vi "FGV Map of Errors.vi"(7 "Operation (Get)":enum16{"Init", "Get", "Update"}(ring)=enum."Get", 8 "error in":errorcluster, 10 "error description":string, 11 "error code":i32) -> (0 "error out":errorcluster, 3 "Custom Errors out":map{i32, string}(c390))   [LabVIEW 2021]
doc: "FGV storing <b>Custom Errors</b> values. Initialize the map by Init <b>Operation</b>, access the map by Get (default) or update the map by selecting Update <b>Operation</b> and wire <b>error code</b> as a key and <b>error description</b> as a value."
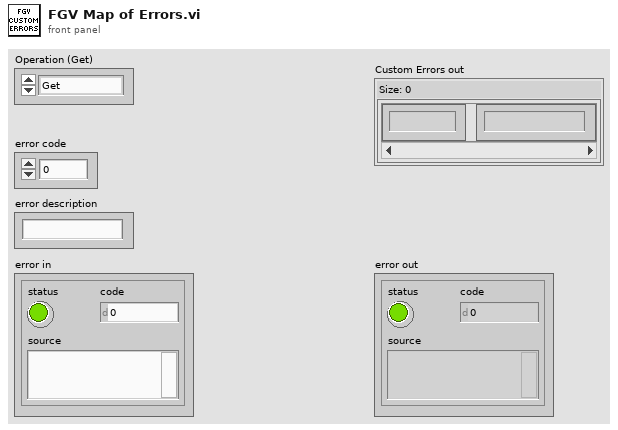
[diagram p1: front panel]
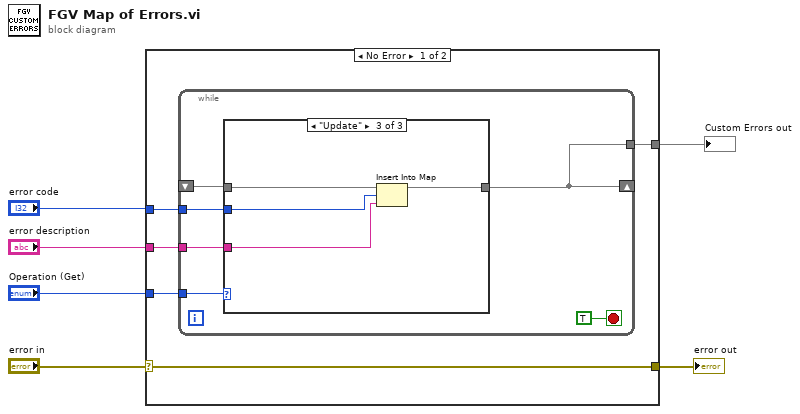
[diagram p0: block diagram]
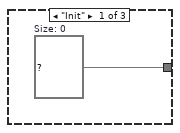
[diagram p2: hidden frame]
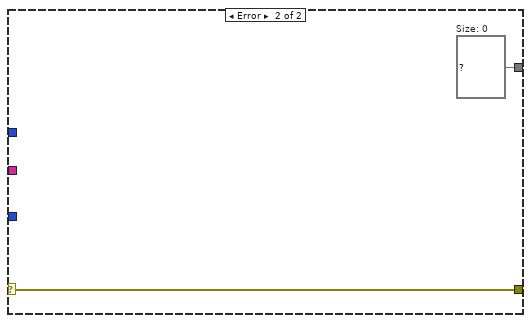
[diagram p4: hidden frame]
diagram:
  n1 = case shown="No Error" "error in" {
    selector: "error in" -> [w11 w25]
    tunnel: [w11 w25] -> w4
    tunnel: "Operation (Get)" -> [w10 _]
    tunnel: [w9 w24] -> w3
    tunnel: "error code" -> [w8 _]
    tunnel: "error description" -> [w7 _]
    frame No Error {
      n2 = while {
        tunnel: w10 -> [w16]
        shift-right: [w14] -> _
        shift-left: _ -> [w15]
        tunnel: [w14] -> w9
        tunnel: w8 -> [w13]
        tunnel: w7 -> [w12]
        stop <- TRUE stop-if-true
        n3 = case shown="\"Update\"" w16 {
          tunnel: w15 -> [_ w19 w22]
          tunnel: [w18 w19 w23] -> w14
          tunnel: w13 -> [_ _ w21]
          tunnel: w12 -> [_ _ w20]
          frame "Init" {
            w18 = map{i32, string} {}  # Size: 0
          }
          frame "Get", Default {
          }
          frame "Update" {
            n4 = Insert Into Map(map in=w22, key=w21, value=w20) -> (map out=w23:map{i32, string})  [unwired: 2 out]
          }
        }
      }
    }
    frame Error {
      w24 = map{i32, string} {}  # Size: 0
    }
  }
  "error out" <- w4
  "Custom Errors out" <- w3
